vi "Write Acceleration.vi"(8 "error in":errorcluster, 10 "Acceleration PVector":refnum<class "PVector.lvclass">, 11 "Mover in":refnum<class "Mover.lvclass">) -> (0 "error out":errorcluster, 3 "Mover out":refnum<class "Mover.lvclass">)   [LabVIEW 2016, in "Mover.lvclass"]
uses:
  Mover.lvclass
  PVector/PVector.lvclass
  Mover.lvclass/Mover.ctl
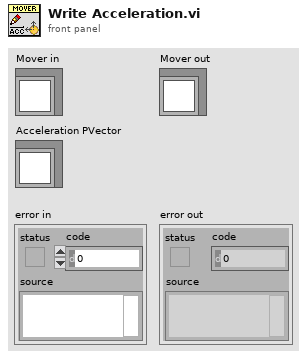
[diagram p1: front panel]
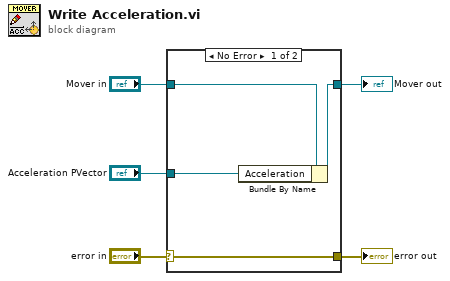
[diagram p0: block diagram]
diagram:
  n1 = case shown="No Error" "error in" {
    selector: "error in" -> [w9 w10]
    tunnel: [w9 w10] -> w4
    tunnel: [w7 w11] -> w2
    tunnel: "Mover in" -> [w8 w11]
    tunnel: "Acceleration PVector" -> [w6 _]
    frame No Error {
      n2 = Bundle By Name(cluster=w8, "Acceleration"=w6) -> (w7:refnum<class "Mover.lvclass">)
    }
    frame Error {
    }
  }
  "error out" <- w4
  "Mover out" <- w2
